vi "Prefix Deps Names for Special Paths.vi"(7 "Prefix to add":string, 8 "error in":errorcluster, 9 "Regex to identify need for prefix":string, 10 "Add Prefix?":bool=TRUE, 11 "Dep Names and Paths":T1) -> (0 "error out":errorcluster, 3 "Prefixed Dep Names and Paths":T1)   [LabVIEW 2018, in "Name and Dependency Processing.lvlib"]
uses:
  Name and Dependency Processing.lvlib
  Dep Names and Paths.ctl
  <vilib>/regexp/Match Regular Expression.xnode
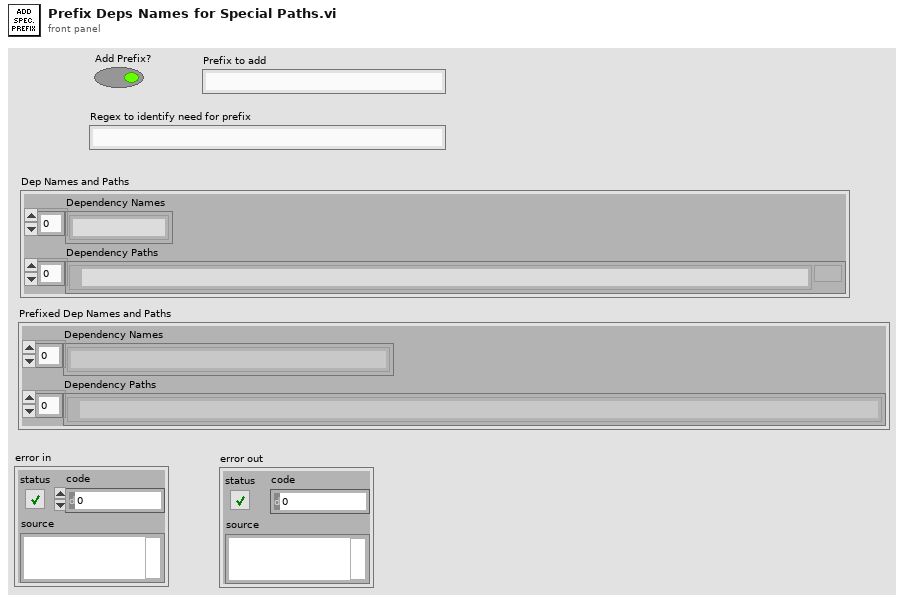
[diagram p1: front panel]
types:
  T1 = typedef "Name and Dependency Processing.lvlib/Dep Names and Paths.ctl" = cluster{"Dependency Names":string[], "Dependency Paths":path[]}
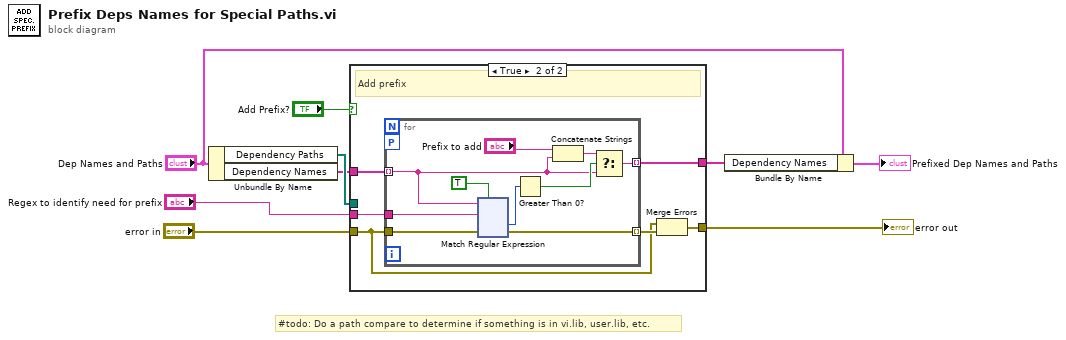
[diagram p0: block diagram]
diagram:
  # "#todo: Do a path compare to determine if something is in vi.lib, user.lib, etc."
  n1 = Unbundle By Name("Dep Names and Paths") -> ("Dependency Paths"=w7:path[], "Dependency Names"=w6:string[])
  n2 = case shown="True" "Add Prefix?" {
    tunnel: w6 -> [w11 w17]
    tunnel: [w11 w16] -> w2
    tunnel: w7 -> [_ _]
    tunnel: "Regex to identify need for prefix" -> [_ w15]
    tunnel: "error in" -> [w10 w12]
    tunnel: [w10 w13] -> w4
    frame False {
      # "Don't add prefix"
    }
    frame True {
      # "Add prefix"
      n3 = for {
        tunnel: w17 -> [w18] mode=indexing
        tunnel: [w27] -> w16 mode=indexing
        workers-P: _ -> [_]
        tunnel: w15 -> [w22]
        tunnel: w12 -> [w20]
        tunnel: [w19] -> w14 mode=indexing
        n4 = xnode "Match Regular Expression"("input string"=w18, "regular expression"=w22, "error in"=w20, "ignore case? (F)"=TRUE) -> ("offset past match"=w25:i32, "error out"=w19:errorcluster)  [unwired: 2 in, 3 out]
        n5 = Greater Than 0?(x=w25) -> (x > 0?=w24:bool)
        n6 = Concatenate Strings("Prefix to add", w18) -> (w26:string)
        n7 = Select(t=w26, s=w24, f=w18) -> (s? t:f=w27:string)
      }
      n8 = Merge Errors(w12, w14) -> (w13:errorcluster)
    }
  }
  "error out" <- w4
  n9 = Bundle By Name(cluster="Dep Names and Paths", "Dependency Names"=w2) -> (→"Prefixed Dep Names and Paths":T1)
